vi "Anlyse Temperature log.vi"(11 "Temperature Log File":path) -> (1 "Test_Finish":timestamp, 2 "Test_Start":timestamp, 3 "Report":string)   [LabVIEW 2024]
uses:
  <vilib>/Utility/NIReport.llb/NI_report.lvclass
  <vilib>/Utility/NIReport.llb/Report Type.ctl
  <vilib>/Utility/NIReport.llb/NI_ReportGenerationCore.lvlib
  <vilib>/Utility/NIReport.llb/Excel/NI_Excel.lvclass
  <vilib>/addons/_office/NI_ReportGenerationToolkit.lvlib
  <vilib>/addons/_office/excel.llb/Excel Get Data ([dbl]).vi
  <vilib>/addons/_office/excel.llb/Excel Get Data ([str]).vi
  <vilib>/Waveform/WDTOps.llb/WDT Get Waveform Subset DBL.vi
panel:
  out "Array":T1(array[cluster])
  out "length":i32
  out "time stamp":timestamp[](array[timestamp])
  out "ReferenceTemperature":dbl[](array[numeric])
  in  "RefChannel":string="3A"
  in  "TopLevel":bool
  out "Array 2":string[](array[string])
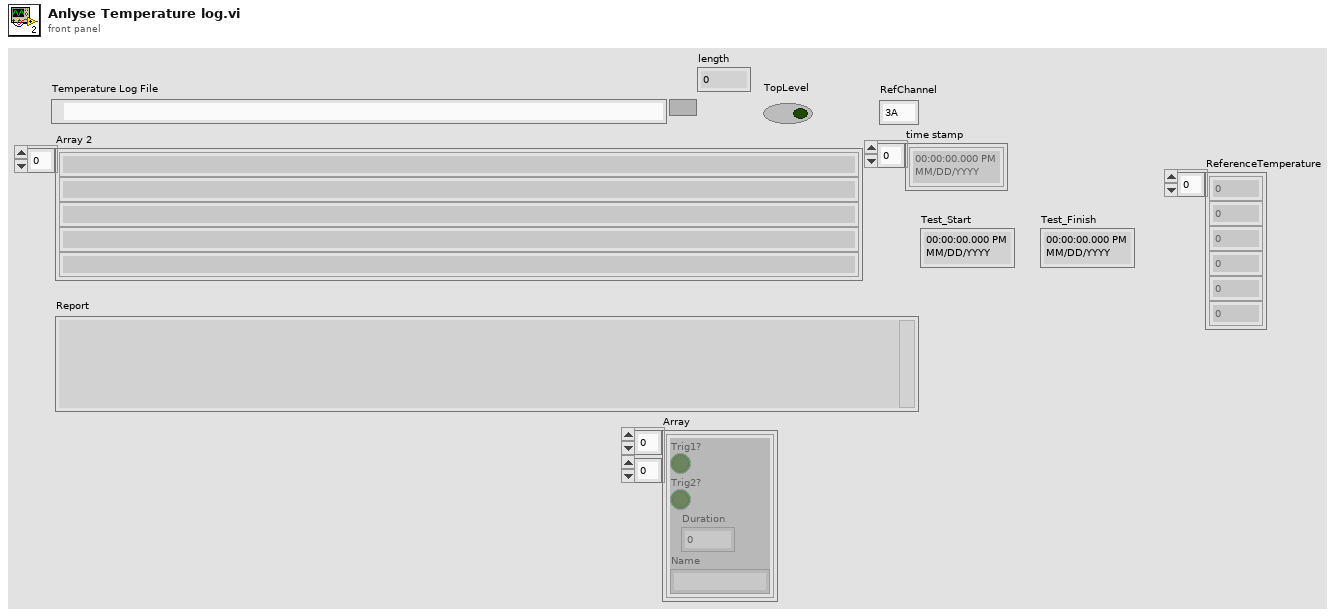
[diagram p1: front panel]
types:
  T1 = cluster{"Trig1?":bool, "Trig2?":bool, "Duration":dbl, "Name":string}[][]
  T2 = typedef "NI_ReportGenerationCore.lvlib/Report Type.ctl" = enum16{"HTML", "Word", "Excel"}
  T3 = cluster{"position (excel)":cluster{"row":i32, "column":i32}, "name (excel)":string, "bookmark (word)":string}
  T4 = cluster{"Trig1?":bool, "Trig2?":bool, "Duration":dbl, "Name":string}[]
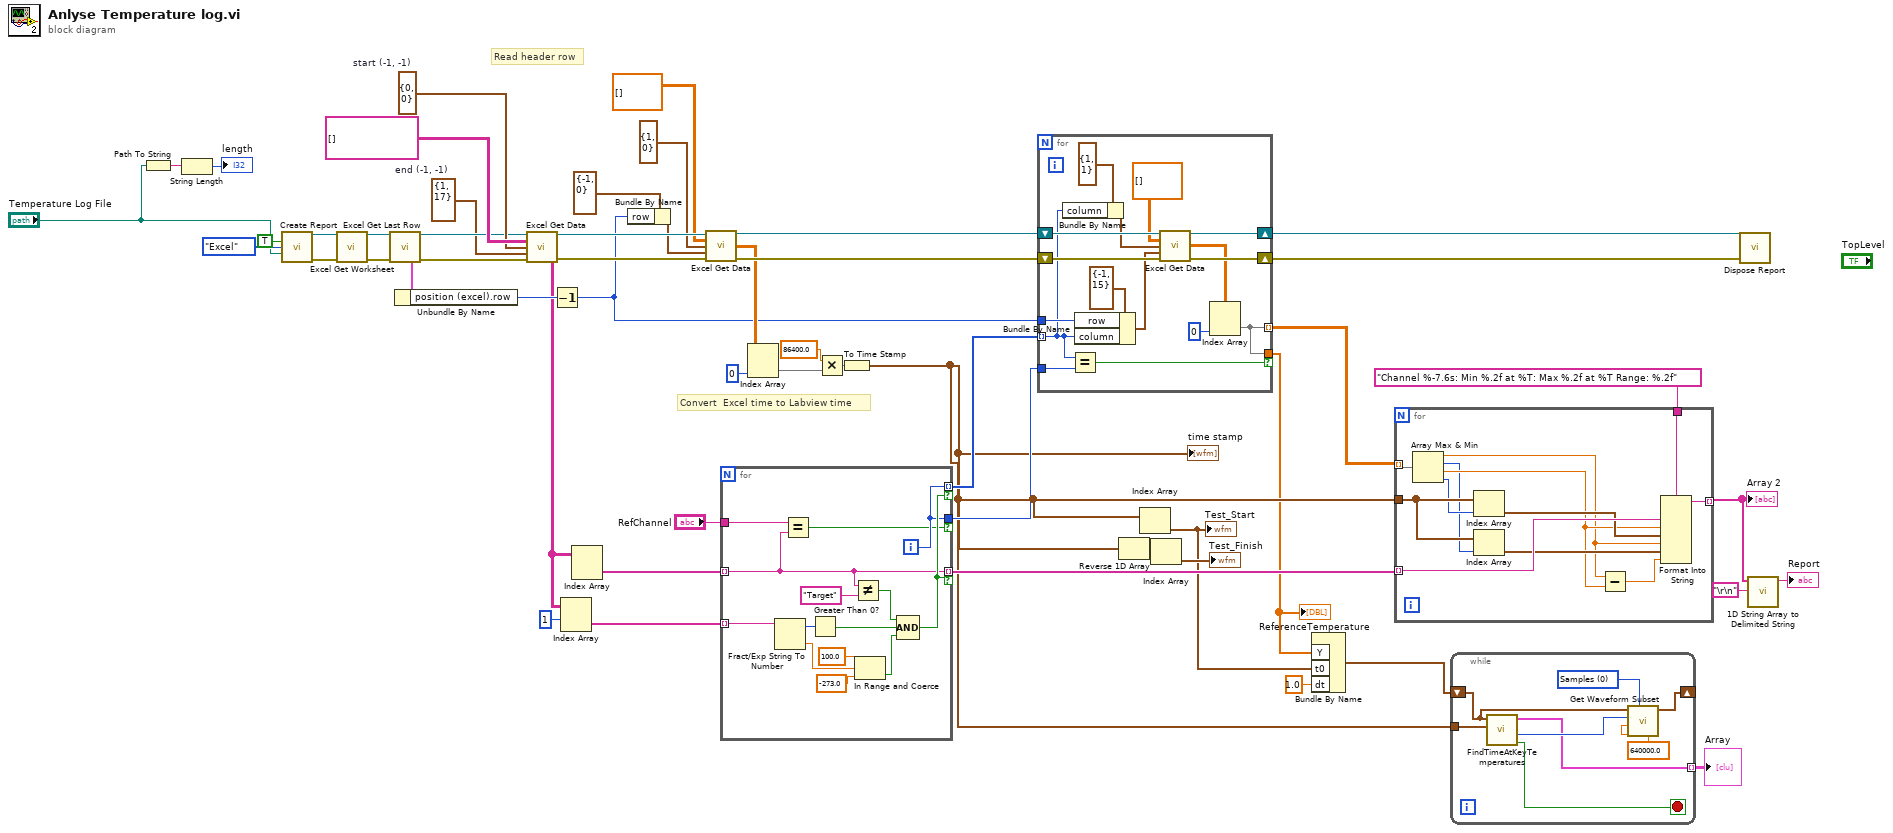
[diagram p0: block diagram]
diagram:
  w41 = cluster{"row":i32, "column":i32} {"row"=1, "column"=17}  # end (-1, -1)
  w49 = cluster{"row":i32, "column":i32} {"row"=0, "column"=0}  # start (-1, -1)
  # "Convert  Excel time to Labview time"
  # "Read header row"
  n1 = Path To String(path="Temperature Log File") -> (string=w9:string)
  n2 = String Length(string=w9) -> (length=→"length":i32)
  n3 = call <vilib>:"Create Report.vi"("display alerts? (F)"=TRUE, "report type"=Report_Type."Excel", "template (empty)"="Temperature Log File") -> ("report out"=w52:refnum<class "NI_report.lvclass">, "error out"=w51:errorcluster)  [unwired: 11 in]
  n4 = call <vilib>:"Excel Get Worksheet.vi"("report in"=w52, "error in (no error)"=w51) -> ("report out"=w45:refnum<class "NI_report.lvclass">, "error out"=w42:errorcluster)  [unwired: 12 in]
  n5 = call <vilib>:"Excel Get Last Row.vi"("report in"=w45, "error in (no error)"=w42) -> ("report out"=w44:refnum<class "NI_report.lvclass">, "MS Office parameters out"=w48:T3, "error out"=w43:errorcluster)  [unwired: 11 in]
  n6 = Unbundle By Name(w48) -> ("position (excel).row"=w27:i32)
  n7 = call-poly <vilib>:"Excel Get Data.vi"("report in"=w44, "data type"=string[][] [], "start (-1, -1)"=w49, "end (-1, -1)"=w41, "error in (no error)"=w43) -> ("report out"=w39:refnum<class "NI_report.lvclass">, "data"=w26:string[][], "error out"=w40:errorcluster)  [unwired: 8 out]
  n8 = Decrement(x=w27) -> (x-1=w18:i32)
  n9 = Index Array(array=w26, index (row)=1) -> (element=w24:string[])  [unwired: 1 in]
  n10 = Index Array(array=w26) -> (element=w23:string[])  [unwired: 2 in]
  n11 = Bundle By Name(cluster=cluster{"row":i32, "column":i32} {"row"=-1, "column"=0} ("end (-1, -1)"), "row"=w18) -> (w33:cluster{"row":i32, "column":i32})
  n12 = call-poly <vilib>:"Excel Get Data.vi"("report in"=w39, "data type"=dbl[][] [], "start (-1, -1)"=cluster{"row":i32, "column":i32} {"row"=1, "column"=0}, "end (-1, -1)"=w33, "error in (no error)"=w40) -> ("report out"=w38:refnum<class "NI_report.lvclass">, "data"=w32:dbl[][], "error out"=w37:errorcluster)  [unwired: 8 out]
  n13 = for {
    tunnel: w24 -> [w67] mode=indexing
    tunnel: w23 -> [w57] mode=indexing
    tunnel: [w57] -> w20 mode=indexing if=w60
    tunnel: [w55] -> w22 mode=indexing if=w60
    tunnel: "RefChannel" -> [w56]
    tunnel: [w55] -> w11 if=w54
    i -> [w55]
    n14 = Fract/Exp String To Number(string=w67) -> (offset past number=w66:i32, number=w64:dbl)  [unwired: 3 in]
    n15 = Equal?(x=w56, y=w57) -> (x = y?=w54:bool)
    n16 = Greater Than 0?(x=w66) -> (x > 0?=w65:bool)
    n17 = Not Equal?(x=w57, y="Target") -> (x != y?=w59:bool)
    n18 = In Range and Coerce(upper limit=100.0, x=w64, lower limit=-273.0) -> (In Range?=w63:bool)  [unwired: 1 out]
    n19 = Compound Arithmetic op=AND(w59, w65, w63) -> (w60:bool)
  }
  n20 = Index Array(array=w32, index (col)=0 ("disabled index (col)")) -> (element=w29:dbl[])  [unwired: 1 in]
  n21 = Multiply(x=86400.0, y=w29) -> (x*y=w31:dbl[])
  n22 = To Time Stamp(1:w31) -> (0:w6:timestamp[])
  "time stamp" <- w6
  n23 = for {
    tunnel: w18 -> [w75]
    shift-right: [w82] -> w46
    shift-left: w38 -> [w81]
    shift-right: [w83] -> w47
    shift-left: w37 -> [w80]
    tunnel: w22 -> [w70] mode=indexing
    tunnel: [w69] -> w21 mode=indexing
    tunnel: w11 -> [w71]
    tunnel: [w69] -> w4 if=w68
    n24 = Bundle By Name(cluster=cluster{"row":i32, "column":i32} {"row"=1, "column"=1} ("start (-1, -1)"), "column"=w70) -> (w74:cluster{"row":i32, "column":i32})
    n25 = Equal?(x=w70, y=w71) -> (x = y?=w68:bool)
    n26 = Bundle By Name(cluster=cluster{"row":i32, "column":i32} {"row"=-1, "column"=15} ("end (-1, -1)"), "row"=w75, "column"=w70) -> (w76:cluster{"row":i32, "column":i32})
    n27 = call-poly <vilib>:"Excel Get Data.vi"("report in"=w81, "data type"=dbl[][] [], "start (-1, -1)"=w74, "end (-1, -1)"=w76, "error in (no error)"=w80) -> ("report out"=w82:refnum<class "NI_report.lvclass">, "data"=w73:dbl[][], "error out"=w83:errorcluster)  [unwired: 8 out]
    n28 = Index Array(array=w73, index (col)=0 ("disabled index (col)")) -> (element=w69:dbl[])  [unwired: 1 in]
  }
  "ReferenceTemperature" <- w4
  n29 = Reverse 1D Array(array=w6) -> (reversed array=w13:timestamp[])
  n30 = Index Array(array=w6) -> (element=w3:timestamp)  [unwired: 1 in]
  "Test_Start" <- w3
  n31 = Index Array(array=w13) -> (element=→"Test_Finish":timestamp)  [unwired: 1 in]
  n32 = Bundle By Name("Y"=w4, "t0"=w3, "dt"=1.0) -> (w2:waveform(dbl))  [unwired: 1 in]
  n33 = for {
    tunnel: w21 -> [w95] mode=indexing
    tunnel: w6 -> [w94]
    tunnel: w20 -> [w93] mode=indexing
    tunnel: [w91] -> w17 mode=indexing
    tunnel: "Channel %-7.6s: Min %.2f at %T: Max %.2f at %T Range: %.2f" ("format string") -> [w90]
    n34 = Array Max & Min(array=w95) -> (max value=w86:dbl, max index (indices)=w84:i32, min value=w87:dbl, min index (indices)=w85:i32)
    n35 = Index Array(array=w94, index=w85) -> (element=w92:timestamp)
    n36 = Index Array(array=w94, index=w84) -> (element=w89:timestamp)
    n37 = Subtract(x=w86, y=w87) -> (x-y=w88:dbl)
    n38 = Format Into String(format string=w90, w93, w87, w92, w86, w89, w88) -> (resulting string=w91:string)  [unwired: 2 in, 1 out]
  }
  "Array 2" <- w17
  n39 = while {
    tunnel: w6 -> [w103]
    shift-right: [w98] -> _
    shift-left: w2 -> [w99]
    tunnel: [w96] -> w1 mode=indexing
    stop <- w97 stop-if-true
    w100 = u16 0 items=["Samples", "Relative Time"] ("start/duration format")
    n40 = call "FindTimeAtKeyTemperatures.vi"("time stamps"=w103, "Temperatures"=w99) -> ("partial?"=w97:bool, "Last Trigger"=w102:i32, "Array"=w96:T4)  [unwired: 7 in]
    n41 = call-poly <vilib>:"Get Waveform Subset.vi"("start/duration format"=w100, "duration"=640000.0, "start samples/time"=w102, "waveform in"=w99) -> ("waveform out"=w98:waveform(dbl))  [unwired: 2 in, 3 out]
  }
  "Array" <- w1
  n42 = call-dynamic "Dispose Report.vi"("report in"=w46, "error in (no error)"=w47) -> ()  [unwired: 13 in, 1 out]
  n43 = call <vilib>:"1D String Array to Delimited String.vi"("delimiter"="\r\n", "string array"=w17) -> ("delimited string"=→"Report":string)  [unwired: 9 in]
